vi "thruster trigger logic.vi"(11 "control":bool) -> (1 "elapsed time":dbl, 3 "signal":bool)   [LabVIEW 2021]
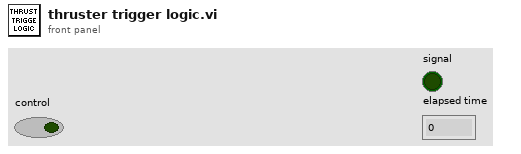
[diagram p1: front panel]
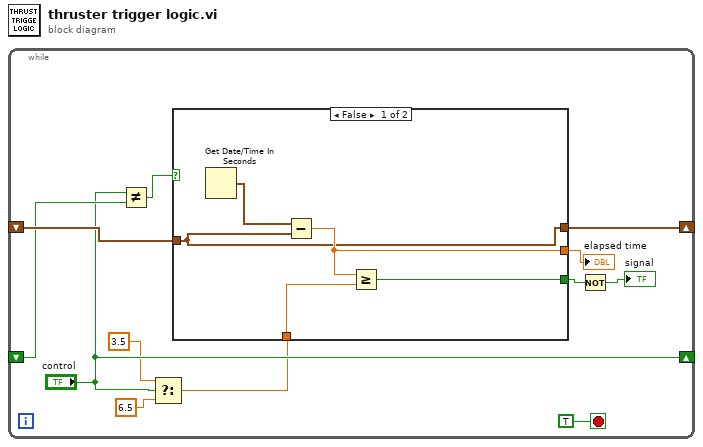
[diagram p0: block diagram]
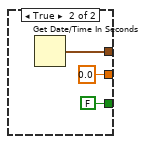
[diagram p2: hidden frame]
diagram:
  n1 = while {
    shift-right: ["control"] -> _
    shift-left: _ -> [w11]
    shift-right: [w8] -> _
    shift-left: _ -> [w12]
    stop <- TRUE stop-if-true
    n2 = Not Equal?(x="control", y=w11) -> (x != y?=w9:bool)
    n3 = Select(t=3.5, s="control", f=6.5) -> (s? t:f=w5:dbl)
    n4 = case shown="False" w9 {
      tunnel: w12 -> [w13 _]
      tunnel: [w13 w20] -> w8
      tunnel: w5 -> [w16 _]
      tunnel: [w15 FALSE] -> w2
      tunnel: [w14 0.0] -> w4
      frame False {
        n5 = Get Date/Time In Seconds() -> (seconds since 1Jan1904=w17:timestamp)
        n6 = Subtract(x=w17, y=w13) -> (x-y=w14:dbl)
        n7 = Greater Or Equal?(x=w14, y=w16) -> (x >= y?=w15:bool)
      }
      frame True {
        n8 = Get Date/Time In Seconds() -> (seconds since 1Jan1904=w20:timestamp)
      }
    }
    "elapsed time" <- w4
    n9 = Not(x=w2) -> (.not. x?=→"signal":bool)
  }
